vi "Degrees and Radians converter.vi"(4 "Units":enum16{"Deg -> Rad", "Rad -> Deg"}(ring), 5 "Angle IN":dbl format="%.2f") -> (2 "Angle Out":dbl format="%.2f")   [LabVIEW 2013]
doc: "Given an angle in degrees or radians, this VI will convert it into the other unit."
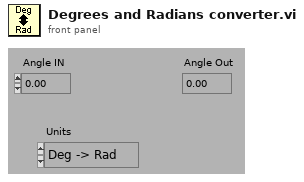
[diagram p1: front panel]
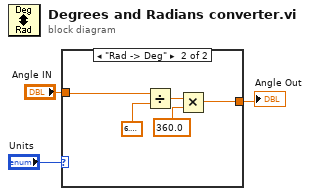
[diagram p0: block diagram]
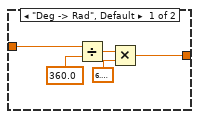
[diagram p2: hidden frame]
diagram:
  n1 = case shown="\"Rad -> Deg\"" "Units" {
    tunnel: "Angle IN" -> [w5 w11]
    tunnel: [w4 w12] -> w1
    frame "Deg -> Rad", Default {
      n2 = Divide(x=w5, y=360.0) -> (x/y=w7:dbl)
      n3 = Multiply(x=w7, y=6.283185307179586) -> (x*y=w4:dbl)
    }
    frame "Rad -> Deg" {
      n4 = Divide(x=w11, y=6.283185307179586) -> (x/y=w13:dbl)
      n5 = Multiply(x=w13, y=360.0) -> (x*y=w12:dbl)
    }
  }
  "Angle Out" <- w1
